vi "onCreateListener.vi"(8 "error in (no error)":errorcluster, 10 "Configuration":refnum<class "Connection.NetworkStream.lvclass">) -> (0 "error out":errorcluster, 3 "Listener":refnum<class "Connection.lvclass">)   [LabVIEW 2013]
uses:
  Connection/Connection.lvclass
  Connection.NetworkStream.lvclass
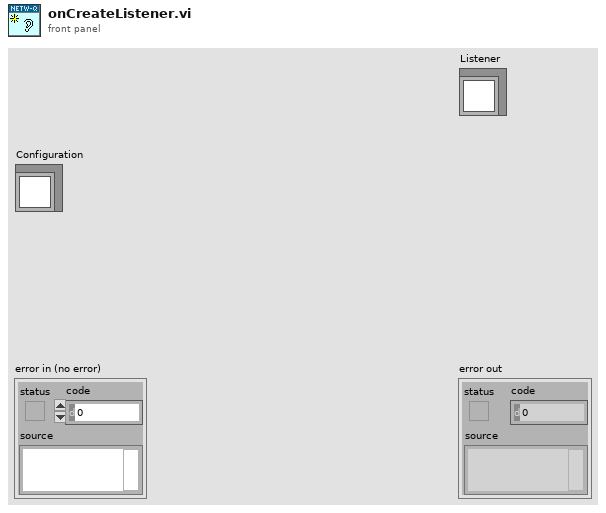
[diagram p1: front panel]
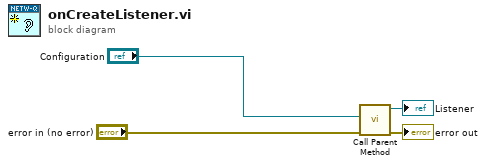
[diagram p0: block diagram]
diagram:
  n1 = call-parent "Call Parent Method"("error in (no error)"="error in (no error)", "Configuration"="Configuration") -> ("error out"=→"error out":errorcluster, "Listener"=→"Listener":refnum<class "Connection.lvclass">)  [unwired: 8 in]
